vi "Act_cmd_2 (SubVI).vi"(4 "W_b [rad/s]":dbl[](array[numeric]), 6 "Euler Angles [rad]":dbl[](array[numeric]), 11 "TVA_cmd [rad]":dbl[](array[numeric])) -> (1 "roll1":dbl, 2 "Act315_Act225":dbl[](array[numeric]))   [LabVIEW 2017]
panel:
  in  "not.Sim_Running":bool
  out "TVA_control_time [s]":dbl
  in  "T [s]":dbl=0.06 format="%#_13g"
  out "roll_angle [rad]":dbl
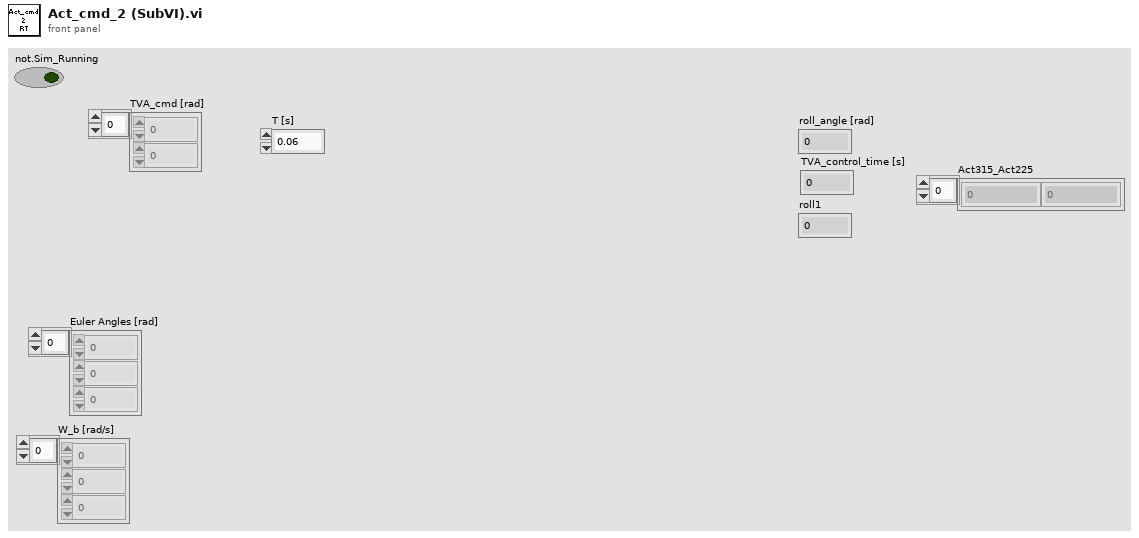
[diagram p1: front panel]
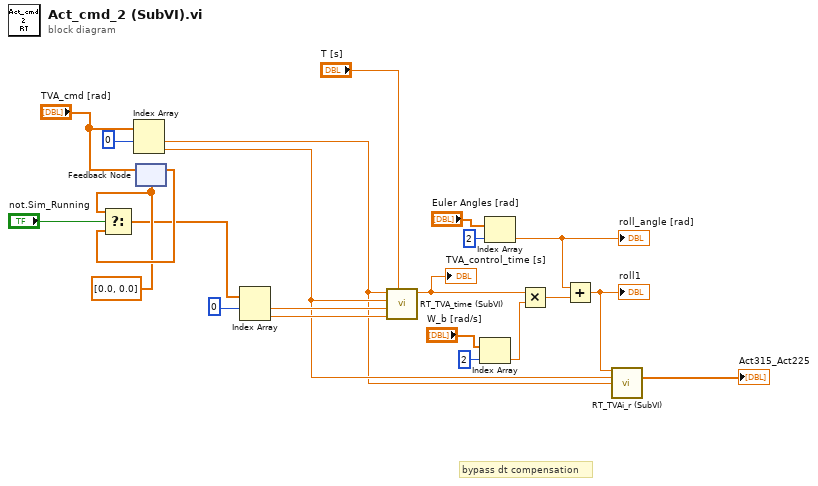
[diagram p0: block diagram]
diagram:
  w5 = dbl[] [0.0, 0.0] ("TVA_cmd")
  # "bypass dt compensation"
  n1 = Index Array(array="TVA_cmd [rad]", index #1=0 ("disabled index (col)")) -> (element #1=w10:dbl, element #2=w11:dbl)  [unwired: 1 in]
  n2 = feedback #1(w5) -> (w6:dbl[])
  n3 = Select(t=w5, s="not.Sim_Running", f=w6) -> (s? t:f=w3:dbl[])
  n4 = feedback-in #1("TVA_cmd [rad]") -> ()
  n5 = Index Array(array=w3, index #1=0 ("disabled index (col)")) -> (element #1=w19:dbl, element #2=w18:dbl)  [unwired: 1 in]
  n6 = call "RT_TVA_time (SubVI).vi"("T [s]"="T [s]", "TVA_y_old"=w18, "TVA_p_old"=w19, "TVA_y"=w11, "TVA_p"=w10) -> ("TVA_control_time [s]"=w9:dbl)  [unwired: 6 in]
  "TVA_control_time [s]" <- w9
  n7 = Index Array(array="W_b [rad/s]", index=2) -> (element=w12:dbl)
  n8 = Index Array(array="Euler Angles [rad]", index=2) -> (element=w8:dbl)
  "roll_angle [rad]" <- w8
  n9 = Multiply(x=w9, y=w12) -> (x*y=w13:dbl)
  n10 = Add(x=w8, y=w13) -> (x+y=w7:dbl)
  "roll1" <- w7
  n11 = call "RT_TVAi_r (SubVI).vi"("roll1"=w7, "TVA_p"=w11, "TVA_y"=w10) -> ("Act315_Act225"=→"Act315_Act225":dbl[])  [unwired: 12 in]
